vi "PH_Powermeter_BaseClass.get data to modify.vi"(0 "i ref in":refnum<vi>, 3 "ms timeout (10000)":i32=10000, 5 "error in (no error)":errorcluster) -> (14 "i ref out":refnum<vi>, 16 "i attribute":T1={"GUI References"={"Head Attributes"=refnum, "Energy"=refnum, "Connection"=refnum, "VISA Resource"=refnum, "Energy evolution"=refnum, "Scaling Factor"=refnum, "Range"=refnum, "Wavelength"=refnum, "Trigger Level"=refnum, "Wanted Settings"=refnum, "Current Settings"=refnum}, "Connection"={"failed checks"=0, "Timeout"=FALSE, "Data read"="", "Failure"=FALSE, "Error"=FALSE, "State"=enum."off"}, "Head Attributes"={"Instrument Type"="", "Head Version"="", "Head Name"="", "Serial Number"="", "Firmware"="", "Sensor Type"="---", "MinimumRange"=0, "Maximum Range"=0, "Min Wavelength"=0, "Max Wavelength"=0}, "VISA resource"="", "Energy"={"current Value"=0.0, "unscaled"=0.0, "Scaling Factor"=0.0}, "Service ID Energy"=-1, "Wanted Settings"={"Trigger Level"=0.0, "Wavelength"=1, "Range"=0}, "Current Settings"={"Trigger Level"=0.0, "Wavelength"=1, "Range"=0}} {"Energy"."unscaled" format="%#_6p"; "Energy"."current Value" format="%#.1p"}, 17 "timed out":bool, 19 "error out":errorcluster)   [LabVIEW 2014, in "PH_Powermeter_BaseClass.lvlib"]
doc: "Reads the attribute data of the object after the access to the data has been locked by the \"acquire\" method. If the attribute data has been locked already, this methods waits until the attribute data is unlocked or there is a timeout.\n\nThe attribute data must be unlocked using the methods \"release\" or \"set modified data\".\n\nLicense Agreement for this software:\n\nCopyright (C)\nGesellschaft für Schwerionenforschung, GSI\nPlanckstr. 1\n64291 Darmstadt\nGermany\n\nContact: D.Beck@gsi.de \n\nThis program is free software; you can redistribute it and/or modify it under the terms of the GNU General Public License as published by the Free Software Foundation; either version 2 of the license, or (at your option) any later version.\n\nThis program is distributed in the hope that it will be useful, but WITHOUT ANY WARRANTY; without even the implied warranty of MERCHANTABILITY or FITNESS FOR A PARTICULAR PURPOSE. See the GNU General License for more details (http://www.gnu.org).\n\nGesellschaft für Schwerionenforschung, GSI\nPlanckstr. 1, 64291 Darmstadt, Germany\nFor all questions and ideas contact: M.Richter@gsi.de, H.Brand@gsi.de or D.Beck@gsi.de.\nLast update: 17-JUN-2004"
uses:
  PH_Powermeter_BaseClass.lvlib
  PH_Powermeter_BaseClass.i attribute.ctl
  PH_Powermeter_BaseClass.GUI Refs.ctl
  PH_Powermeter_BaseClass.Head Attributes.ctl
  PH_Powermeter_BaseClass.Energy.ctl
  PH_Powermeter_BaseClass.Connection.ctl
  PH_Powermeter_BaseClass.State.ctl
  PH_gentec_BaseClass.Head Settings.ctl
  CS_Core/CSObj/CSObj.lvlib
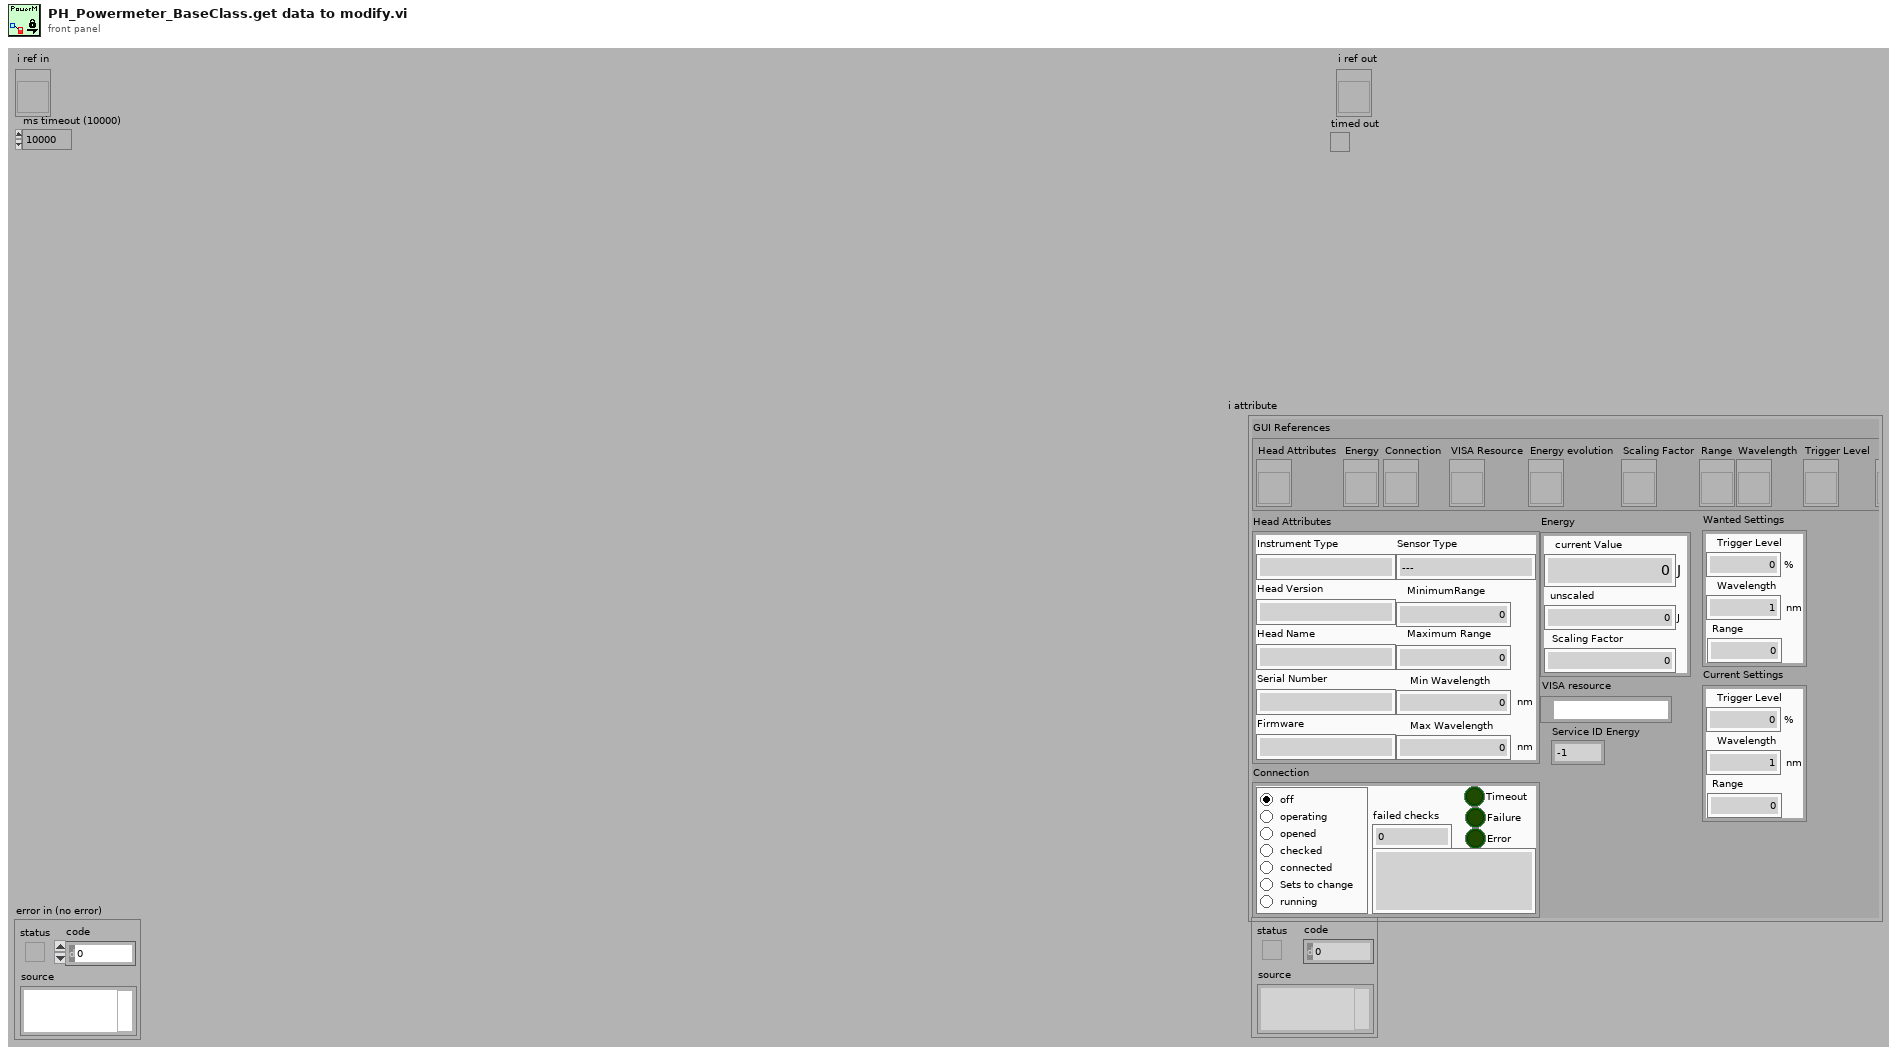
[diagram p1: front panel]
types:
  T1 = typedef "PH_Powermeter_BaseClass.lvlib/PH_Powermeter_BaseClass.i attribute.ctl" = cluster{"GUI References":T2, "Connection":T3, "Head Attributes":T5, "VISA resource":refnum<visa-resource-name>, "Energy":T6, "Service ID Energy":i32, "Wanted Settings":T7, "Current Settings":T7}
  T2 = typedef "PH_Powermeter_BaseClass.lvlib/PH_Powermeter_BaseClass.GUI Refs.ctl" = cluster{"Head Attributes":refnum<vi>, "Energy":refnum<vi>, "Connection":refnum<vi>, "VISA Resource":refnum<vi>, "Energy evolution":refnum<vi>, "Scaling Factor":refnum<vi>, "Range":refnum<vi>, "Wavelength":refnum<vi>, "Trigger Level":refnum<vi>, "Wanted Settings":refnum<vi>, "Current Settings":refnum<vi>}
  T3 = typedef "PH_Powermeter_BaseClass.lvlib/PH_Powermeter_BaseClass.Connection.ctl" = cluster{"failed checks":i8, "Timeout":bool, "Data read":string, "Failure":bool, "Error":bool, "State":T4}
  T4 = typedef "PH_Powermeter_BaseClass.lvlib/PH_Powermeter_BaseClass.State.ctl" = enum32{"off", "operating", "opened", "checked", "connected", "Sets to change", "running"}
  T5 = typedef "PH_Powermeter_BaseClass.lvlib/PH_Powermeter_BaseClass.Head Attributes.ctl" = cluster{"Instrument Type":string, "Head Version":string, "Head Name":string, "Serial Number":string, "Firmware":string, "Sensor Type":string, "MinimumRange":u32, "Maximum Range":u32, "Min Wavelength":i32, "Max Wavelength":i32}
  T6 = typedef "PH_Powermeter_BaseClass.lvlib/PH_Powermeter_BaseClass.Energy.ctl" = cluster{"current Value":dbl, "unscaled":dbl, "Scaling Factor":dbl}
  T7 = typedef "PH_Powermeter_BaseClass.lvlib/PH_gentec_BaseClass.Head Settings.ctl" = cluster{"Trigger Level":dbl, "Wavelength":u32, "Range":u32}
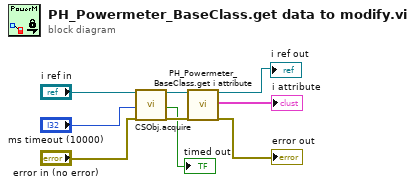
[diagram p0: block diagram]
diagram:
  n1 = call "CSObj.acquire.vi"("i ref in"="i ref in", "ms timeout (10000)"="ms timeout (10000)", "error in (no error)"="error in (no error)") -> ("i ref out"=w8:refnum<vi>, "timed out"=→"timed out":bool, "error out"=w5:errorcluster)  [unwired: 14 in]
  n2 = call "PH_Powermeter_BaseClass.get i attribute.vi"("i ref in"=w8, "error in (no error)"=w5) -> ("i ref out"=→"i ref out":refnum<vi>, "i attribute"=→"i attribute":T1, "error out"=→"error out":errorcluster)  [unwired: 15 in]
